vi "StudentScope - Save to Disk.vi"(2 "Y Values":dbl[][](array[numeric]), 3 "Rate":dbl) -> (0 "error out":errorcluster)   [LabVIEW 2015]
uses:
  Instance           1 35Saved   StudentScope - Save to Disk .vi
  Instance           2 35Saved   StudentScope - Save to Disk .vi
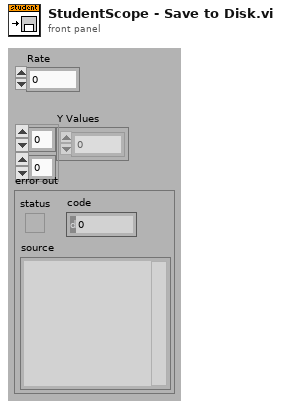
[diagram p1: front panel]
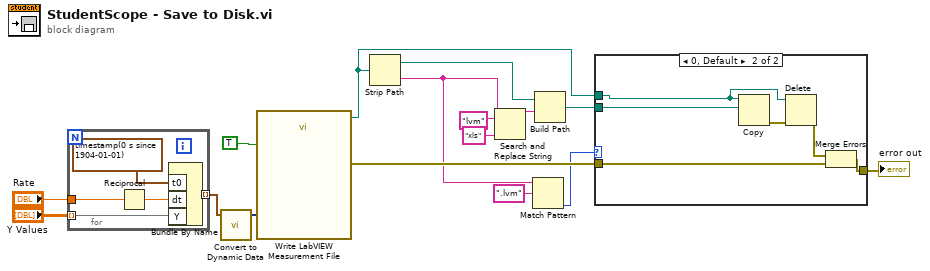
[diagram p0: block diagram]
diagram:
  n1 = for {
    tunnel: "Rate" -> [w17]
    tunnel: "Y Values" -> [w20] mode=indexing
    tunnel: [w19] -> w16 mode=indexing
    n2 = Reciprocal(x=w17) -> (1/x=w18:dbl)
    n3 = Bundle By Name("t0"=timestamp(0 s since 1904-01-01), "dt"=w18, "Y"=w20) -> (w19:waveform(dbl))  [unwired: 1 in]
  }
  n4 = call "Convert to Dynamic Data"("Array of Waveforms"=w16) -> ("Dynamic Data Type"=w13:dynamicdata)  [unwired: 3 in]
  n5 = call "Write LabVIEW Measurement File"("Reset"=TRUE, "Signals"=w13) -> ("error out"=w11:errorcluster, "File Name Out"=w2:path)  [unwired: 7 in, 1 out]
  n6 = Strip Path(path=w2) -> (stripped path=w1:path, name=w4:string)
  n7 = Search and Replace String(input string=w4, search string="lvm", replace string="xls" ("replace string (\"\")")) -> (result string=w8:string)  [unwired: 5 in, 3 out]
  n8 = Match Pattern(string=w4, regular expression=".lvm") -> (offset past match=w9:i32)  [unwired: 1 in, 3 out]
  n9 = Build Path(base path=w1, name or relative path=w8) -> (appended path=w5:path)
  n10 = case shown="0, Default" w9 {
    tunnel: w11 -> [w22 w23]
    tunnel: [w22 w28] -> w10
    tunnel: w5 -> [_ w25]
    tunnel: w2 -> [_ w24]
    frame -1 {
    }
    frame 0, Default {
      n11 = Copy(10:w25, 11:w24) -> (0:w27:errorcluster)  [unwired: 3 in, 2 out]
      n12 = Delete(path (use dialog)=w24, error in=w27) -> (error out=w26:errorcluster)  [unwired: 3 in, 2 out]
      n13 = Merge Errors(w26, w23) -> (w28:errorcluster)
    }
  }
  "error out" <- w10
